vi "Untitled 7.vi"(8 "error in (no error)":errorcluster) -> (0 "error out":errorcluster)   [LabVIEW 2017, in "LibraryGcode.lvlib" / "QueueClass.lvclass"]
uses:
  QueueClass.lvclass
  control/UartCmdQueueUpdate.ctl
  control/Queue/TypeDataPOS.ctl
panel:
  out "output cluster":refnum<class "QueueClass.lvclass">
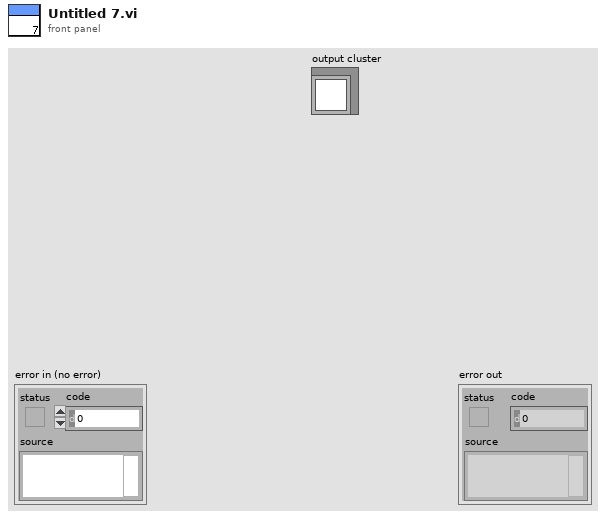
[diagram p1: front panel]
types:
  T1 = typedef "TypeDataPOS.ctl" = cluster{"Command":T2, "POS":cluster{"X":dbl, "Y":dbl, "Z":dbl}, "DEGREES":cluster{"X":dbl, "Y":dbl}}
  T2 = typedef "UartCmdQueueUpdate.ctl" = enum16{"updatePos", "UpdateConfigAccel", "UpdateConfigFeed", "UpdateConfigUnit", "UpdateConfigStartAccel"}
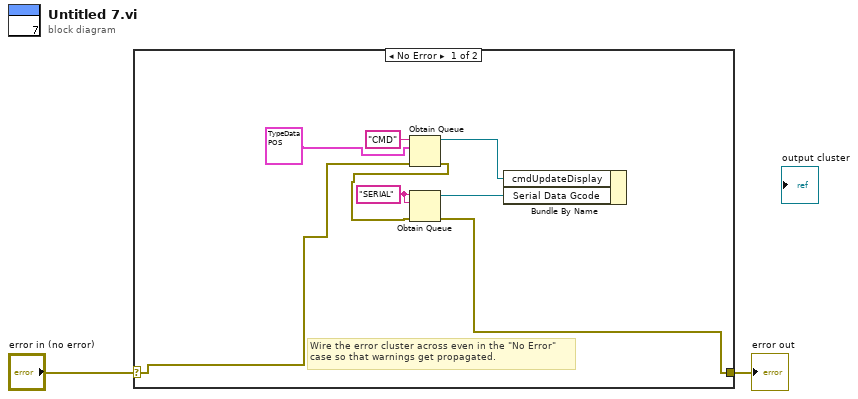
[diagram p0: block diagram]
diagram:
  n1 = case shown="No Error" "error in (no error)" {
    selector: "error in (no error)" -> [w9 w11]
    tunnel: [w7 w11] -> w1
    frame No Error {
      w3 = "SERIAL" ("name (unnamed)")
      # "Wire the error cluster across even in the \"No Error\"\ncase so that warnings get propagated."
      n2 = Obtain Queue(name (unnamed)="CMD", element data type=T1 {"Command"=enum."updatePos", "POS"={"X"=0.0, "Y"=0.0, "Z"=0.0}, "DEGREES"={"X"=0.0, "Y"=0.0}} ("TypeDataPOS"), error in (no error)=w9) -> (queue out=w6:refnum<queue>, error out=w8:errorcluster)  [unwired: 2 in, 1 out]
      n3 = Obtain Queue(name (unnamed)=w3, element data type=w3, error in (no error)=w8) -> (queue out=w5:refnum<queue>, error out=w7:errorcluster)  [unwired: 2 in, 1 out]
      n4 = Bundle By Name("cmdUpdateDisplay"=w6, "Serial Data Gcode"=w5) -> ()  [unwired: 1 in, 1 out]
    }
    frame Error {
    }
  }
  "error out" <- w1
